vi "LabVIEW Main Application.vi"() -> ()   [LabVIEW 2019]
uses:
  <vilib>/numeric/Random Number (Range) DBL.vi
panel:
  out "Error Out":errorcluster
  in  "Error In":errorcluster
  in  "Exit Button":bool
  out "Celsius":dbl(slide)=11.110537127479736 caption="Celsius:" scale=10.0..30.0
  out "Fahrenheit":dbl(slide)=51.99896682946353 caption="Fahrenheit:" scale=0.0..100.0
  in  "New Sensor Button":bool
  in  "SensorList":i32(listbox)=-1 caption="Sensor List:"
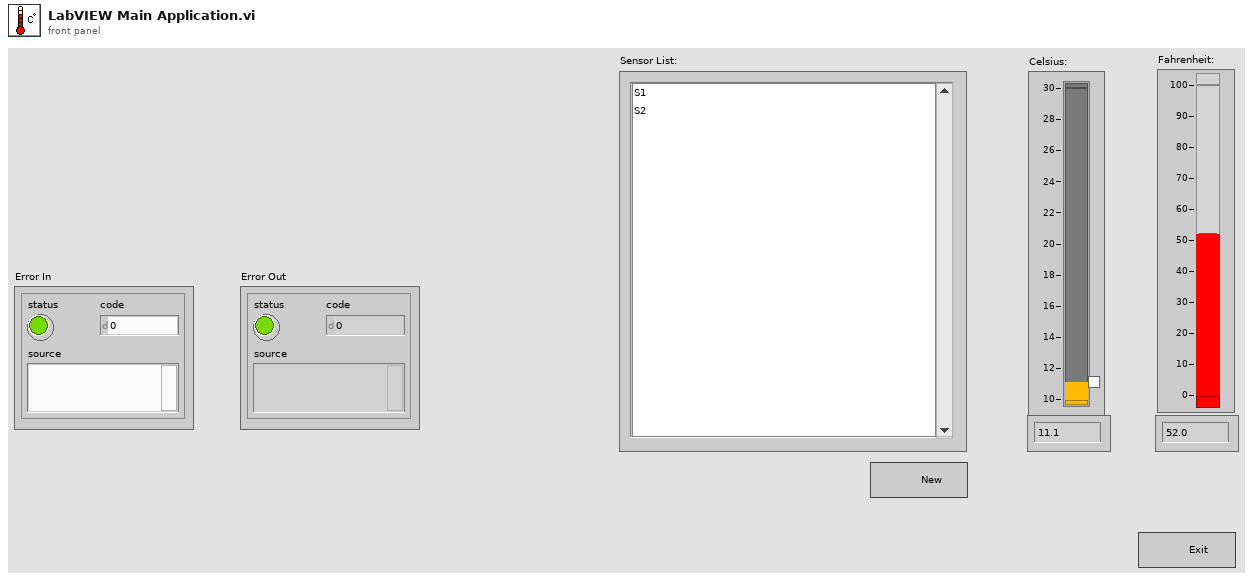
[diagram p1: front panel]
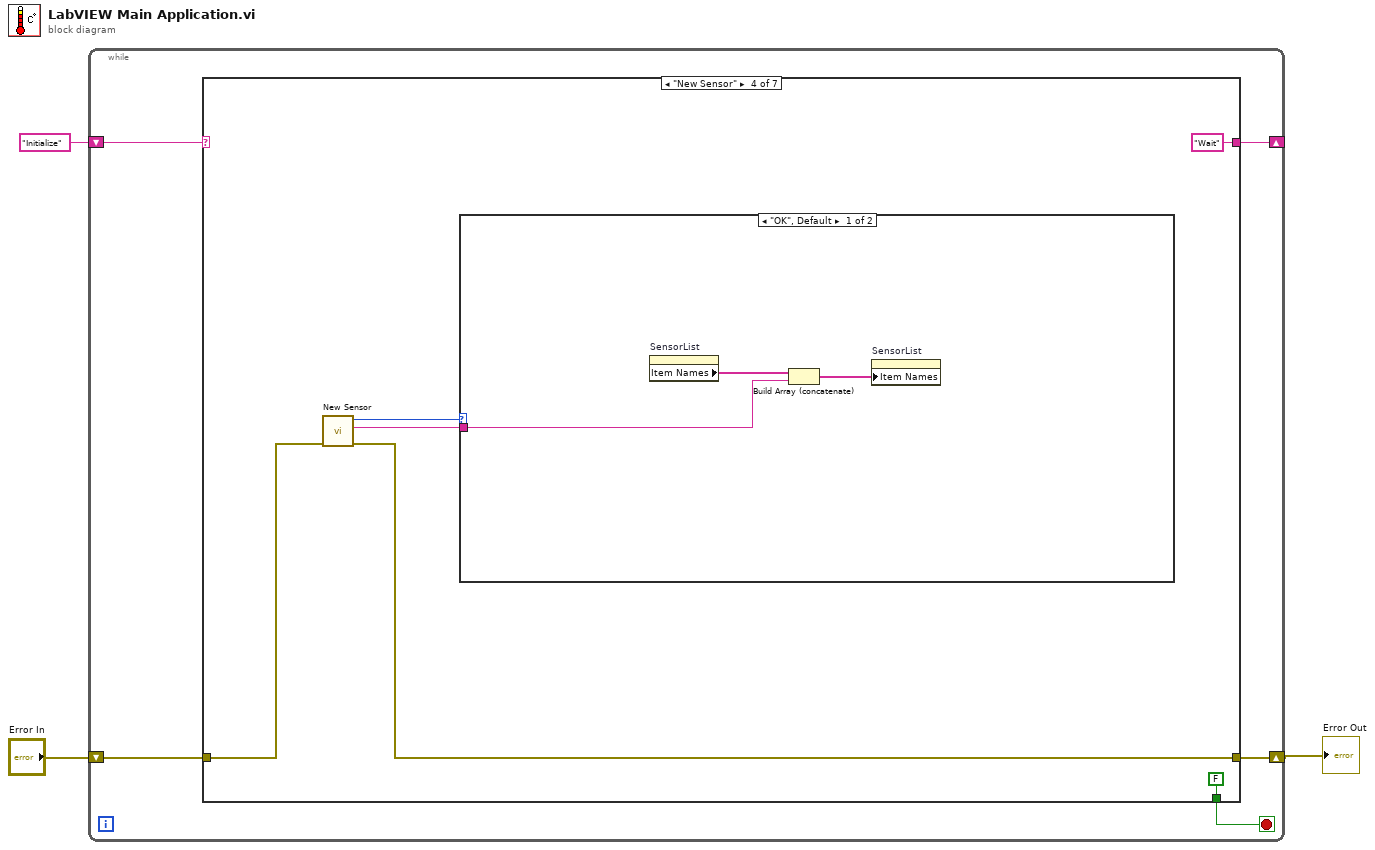
[diagram p0: block diagram]
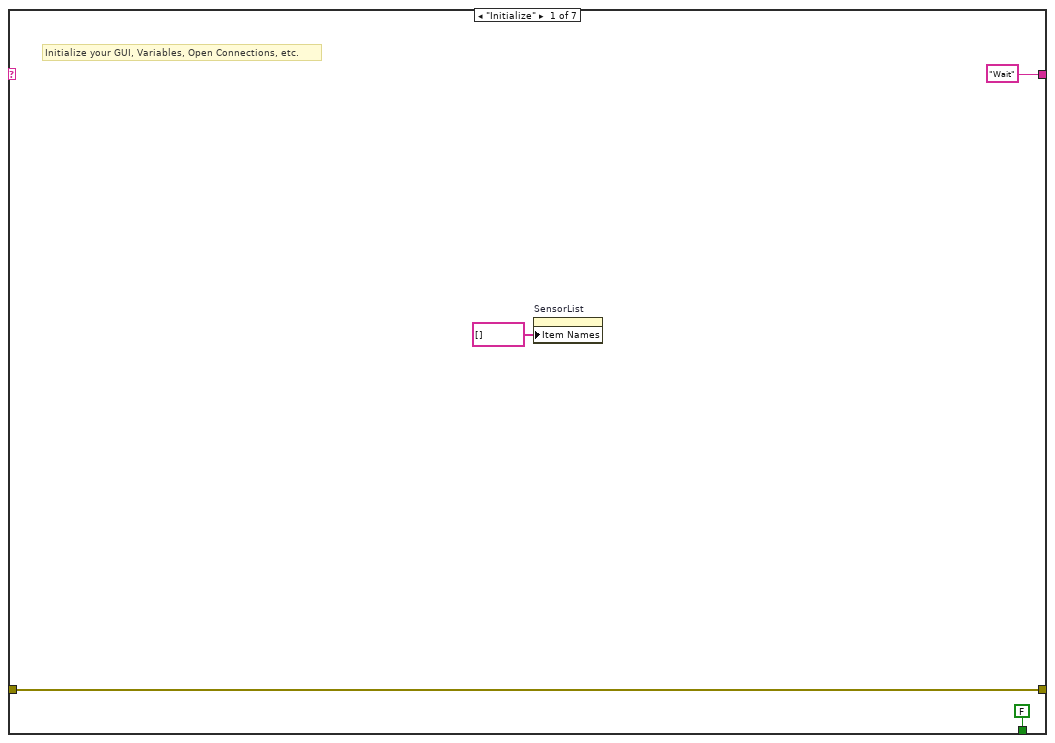
[diagram p2: hidden frame]
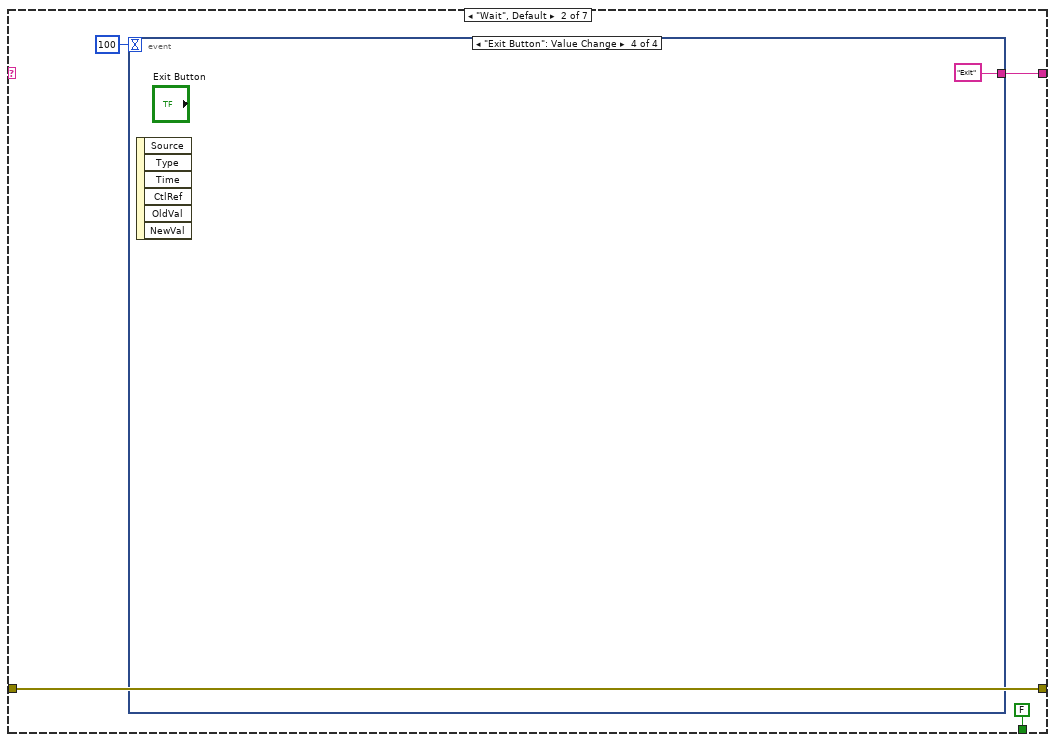
[diagram p3: hidden frame]
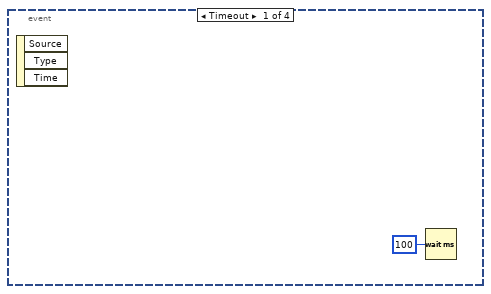
[diagram p4: hidden frame]
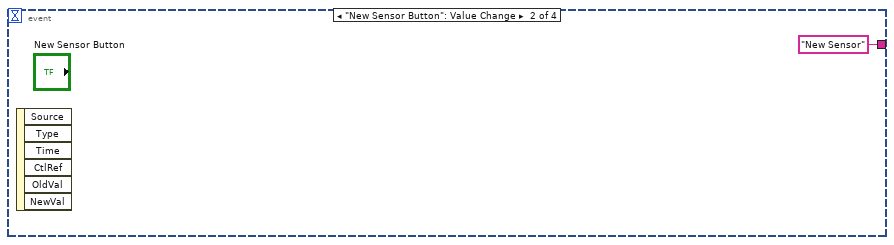
[diagram p5: hidden frame]
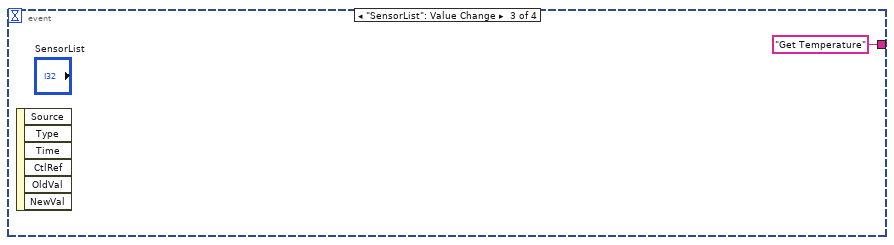
[diagram p6: hidden frame]
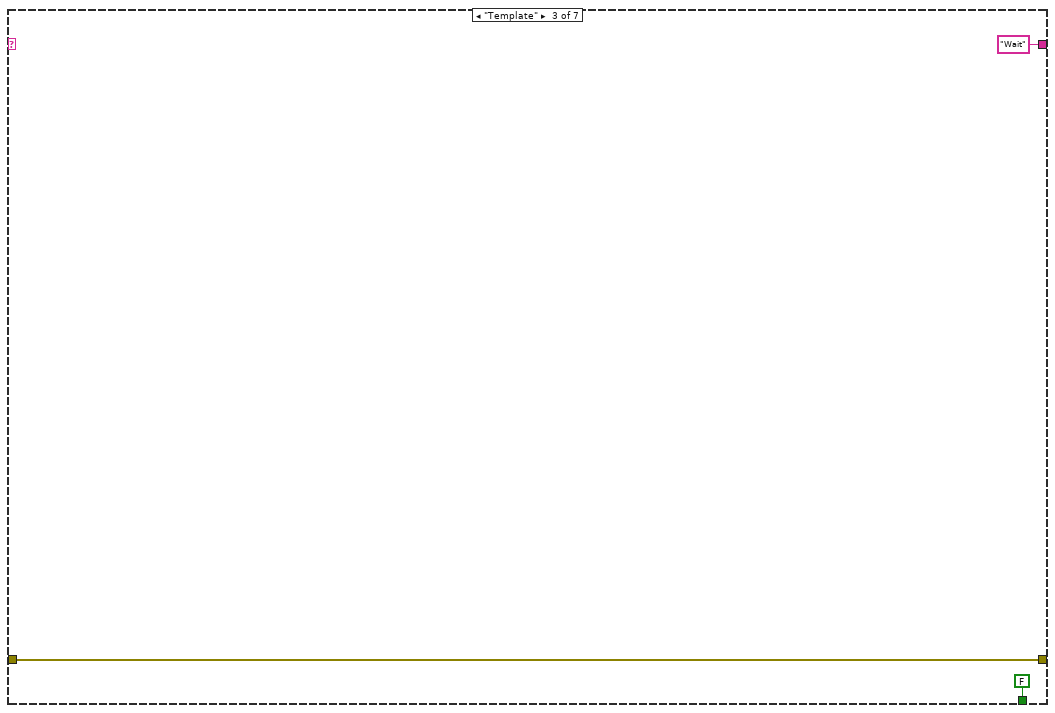
[diagram p7: hidden frame]
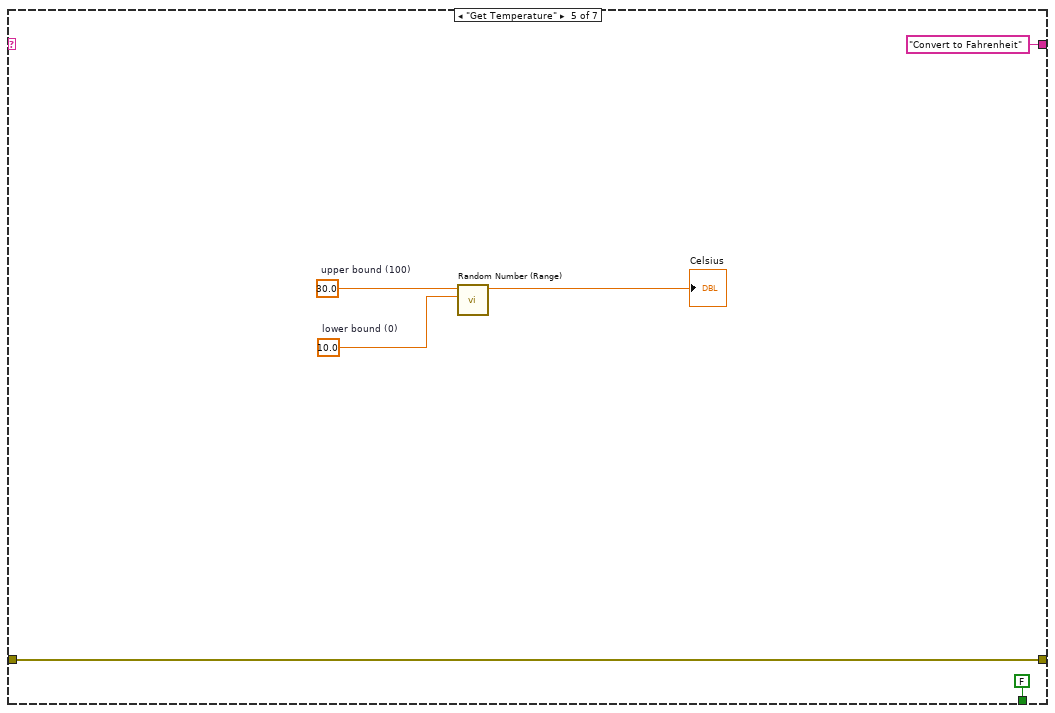
[diagram p9: hidden frame]
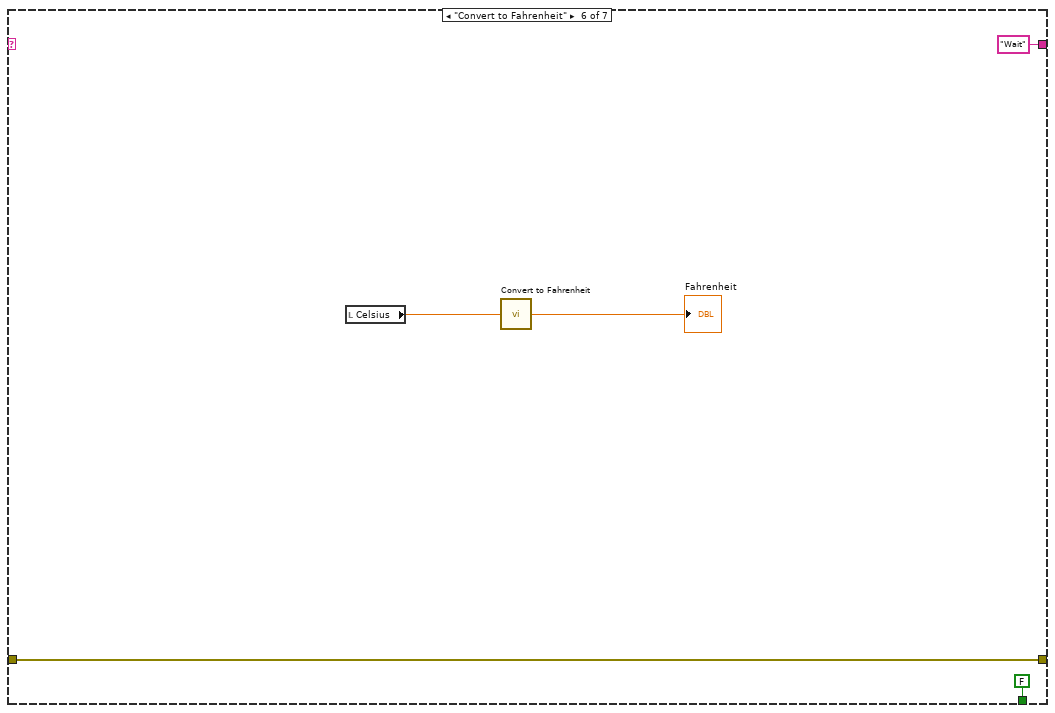
[diagram p10: hidden frame]
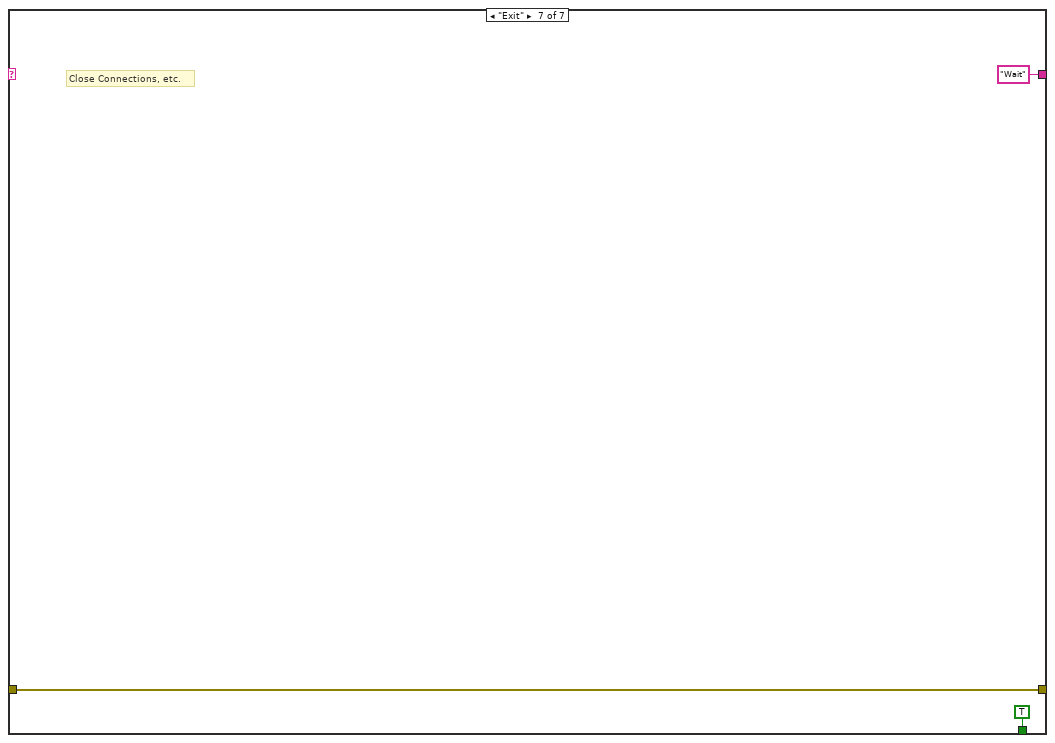
[diagram p11: hidden frame]
diagram:
  n1 = while {
    shift-right: [w7] -> _
    shift-left: "Initialize" -> [w8]
    shift-right: [w4] -> w1
    shift-left: "Error In" -> [w5]
    stop <- w6 stop-if-true
    n2 = case shown="\"New Sensor\"" w8 {
      tunnel: ["Wait" w14 "Wait" "Wait" "Convert to Fahrenheit" "Wait" "Wait"] -> w7
      tunnel: [FALSE FALSE FALSE FALSE FALSE FALSE TRUE] -> w6
      tunnel: [w10 w13 w21 w27 w36 w41 w44] -> w4
      tunnel: w5 -> [w10 w13 w21 w26 w36 w41 w44]
      frame "Initialize" {
        # "Initialize your GUI, Variables, Open Connections, etc."
        n3 = property on="SensorList" class="LstBox (strict)"("Item Names"=string[] []) -> ()  [unwired: 2 in, 2 out]
      }
      frame "Wait", Default {
        n4 = event shown="[3] \"Exit Button\": Value Change" {
          selector: _ -> [_ _ _ _]
          dyn-events: _ -> [_ _ _ _]
          timeout: 100 -> [_ _ _ _]
          tunnel: [_ "New Sensor" "Get Temperature" "Exit"] -> w14
          event Timeout {
            n5 = event-data() -> ()  [unwired: 1 in, 3 out]
            n6 = Wait (ms)(milliseconds to wait=u32 100) -> ()  [unwired: 1 out]
          }
          event "New Sensor Button": Value Change {
            n7 = event-data() -> ()  [unwired: 1 in, 6 out]
          }
          event "SensorList": Value Change {
            n8 = event-data() -> ()  [unwired: 1 in, 6 out]
          }
          event "Exit Button": Value Change {
            n9 = event-data() -> ()  [unwired: 1 in, 6 out]
          }
        }
      }
      frame "Template" {
      }
      frame "New Sensor" {
        n10 = call "New Sensor.vi"("Error In"=w26) -> ("Error Out"=w27:errorcluster, "SensorName Out"=w24:string, "Status"=w25:enum16{"OK", "Cancel"})  [unwired: 8 in]
        n11 = case shown="\"OK\", Default" w25 {
          tunnel: w24 -> [w31 _]
          frame "OK", Default {
            n12 = property on="SensorList" class="LstBox (strict)"() -> ("Item Names"=w32:string[])  [unwired: 2 in, 2 out]
            n13 = Build Array (concatenate)(w32, w31) -> (w30:string[])
            n14 = property on="SensorList" class="LstBox (strict)"("Item Names"=w30) -> ()  [unwired: 2 in, 2 out]
          }
          frame "Cancel" {
          }
        }
      }
      frame "Get Temperature" {
        w34 = 10.0  # lower bound (0)
        w35 = 30.0  # upper bound (100)
        n15 = call-poly <vilib>:"Random Number (Range).vi"("lower bound (0)"=w34, "upper bound (100)"=w35) -> ("number"=→"Celsius":dbl)  [unwired: 9 in]
      }
      frame "Convert to Fahrenheit" {
        n16 = local read "Celsius"() -> (w40:dbl)
        n17 = call "Convert to Fahrenheit.vi"("Celsius"=w40) -> ("Fahrenheit"=→"Fahrenheit":dbl)
      }
      frame "Exit" {
        # "Close Connections, etc."
      }
    }
  }
  "Error Out" <- w1
